vi "Write COM SELECTED NXP.vi"(8 "error in (no error)":errorcluster, 10 "COM SELECTED":refnum<visa-resource-name>, 11 "NXP in":refnum<class "NXP.lvclass">) -> (0 "error out":errorcluster, 3 "NXP out":refnum<class "NXP.lvclass">)   [LabVIEW 2019, in "NXP.lvclass"]
uses:
  NXP.lvclass
  NXP.lvclass/NXP.ctl
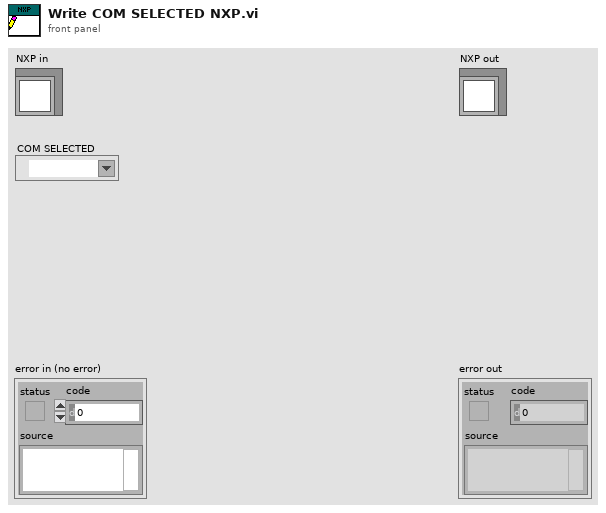
[diagram p1: front panel]
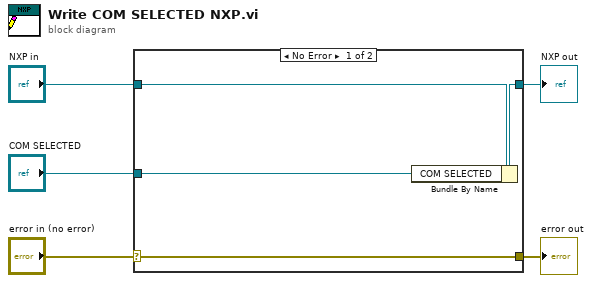
[diagram p0: block diagram]
diagram:
  n1 = case shown="No Error" "error in (no error)" {
    selector: "error in (no error)" -> [w9 w10]
    tunnel: [w9 w10] -> w4
    tunnel: [w7 w11] -> w2
    tunnel: "NXP in" -> [w8 w11]
    tunnel: "COM SELECTED" -> [w6 _]
    frame No Error {
      n2 = Bundle By Name(cluster=w8, "COM SELECTED"=w6) -> (w7:refnum<class "NXP.lvclass">)
    }
    frame Error {
    }
  }
  "error out" <- w4
  "NXP out" <- w2
